vi "Controller VI.vi"(6 "Current Time In":u32, 7 "Read String":string, 8 "Down Detect Time In":u32, 9 "Up Detect Time In":u32, 10 "Left Detect Time In":u32, 11 "Right Detect Time In":u32) -> (0 "Down Detect Time Out":u32, 1 "Up Detect Time Out":u32, 2 "Left Detect Time Out":u32, 3 "Right detect Time Out":u32, 4 "Control Cluster":T1 {"Yaw Speed" scale=-1.0..1.0; "Vertical Speed" scale=-1.0..1.0; "Pitch" scale=-1.0..1.0; "Roll" scale=-1.0..1.0}, 5 "Command string":string)   [LabVIEW 2014]
uses:
  Others/Control cluster.ctl
  Global.vi
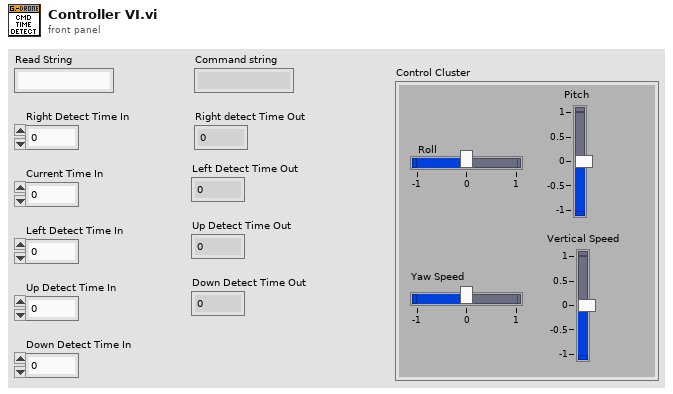
[diagram p1: front panel]
types:
  T1 = typedef "Control cluster.ctl" = cluster{"Roll":sgl, "Pitch":sgl, "Vertical Speed":sgl, "Yaw Speed":sgl}
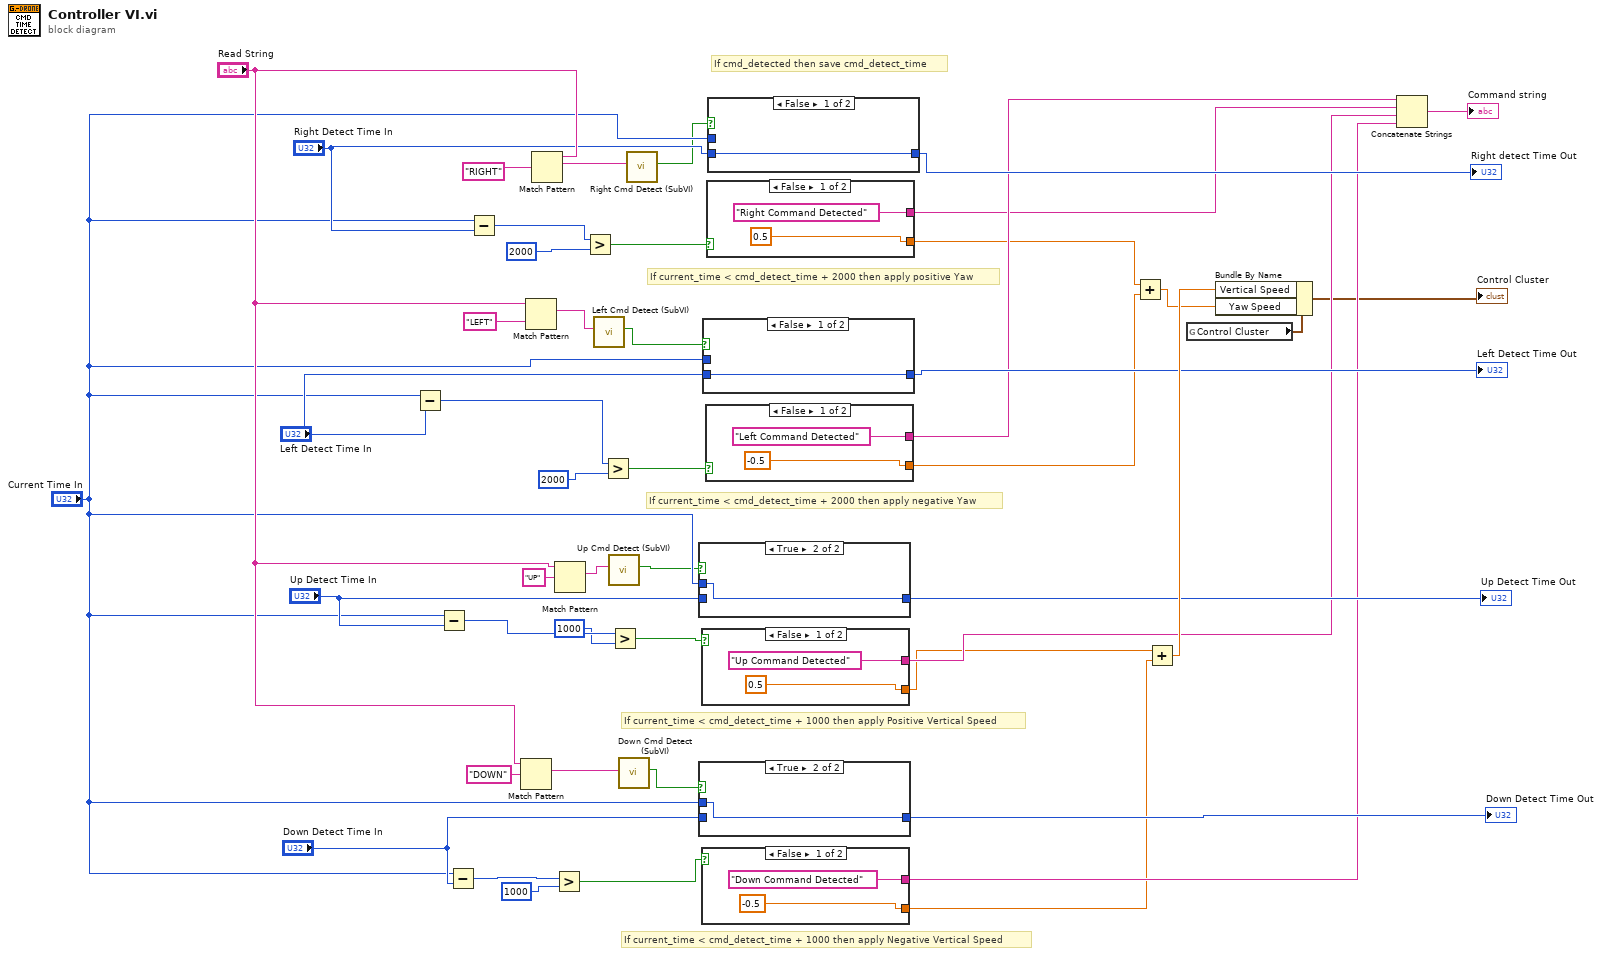
[diagram p0: block diagram]
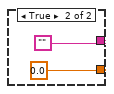
[diagram p2: hidden frame]
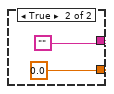
[diagram p4: hidden frame]
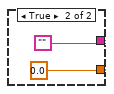
[diagram p6: hidden frame]
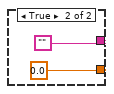
[diagram p8: hidden frame]
diagram:
  # "If current_time < cmd_detect_time + 1000 then apply Negative Vertical Speed"
  # "If current_time < cmd_detect_time + 1000 then apply Positive Vertical Speed"
  # "If current_time < cmd_detect_time + 2000 then apply negative Yaw"
  # "If cmd_detected then save cmd_detect_time"
  # "If current_time < cmd_detect_time + 2000 then apply positive Yaw"
  n1 = Subtract(x="Current Time In", y="Left Detect Time In") -> (x-y=w11:u32)
  n2 = Subtract(x="Current Time In", y="Up Detect Time In") -> (x-y=w19:u32)
  n3 = Subtract(x="Current Time In", y="Down Detect Time In") -> (x-y=w27:u32)
  n4 = Subtract(x="Current Time In", y="Right Detect Time In") -> (x-y=w3:u32)
  n5 = Match Pattern(string="Read String", regular expression="DOWN") -> (match substring=w31:string)  [unwired: 1 in, 3 out]
  n6 = Match Pattern(string="Read String", regular expression="LEFT") -> (match substring=w8:string)  [unwired: 1 in, 3 out]
  n7 = Match Pattern(string="Read String", regular expression="RIGHT") -> (match substring=w17:string)  [unwired: 1 in, 3 out]
  n8 = Greater?(x=w27, y=u32 1000) -> (0:w29:bool)
  n9 = Match Pattern(string="Read String", regular expression="UP") -> (match substring=w21:string)  [unwired: 1 in, 3 out]
  n10 = Greater?(x=w3, y=u32 2000) -> (0:w2:bool)
  n11 = call "Left Cmd Detect (SubVI).vi"("Read String"=w8) -> ("Left Command"=w9:bool)  [unwired: 10 in]
  n12 = Greater?(x=w11, y=u32 2000) -> (0:w12:bool)
  n13 = call "Up Cmd Detect (SubVI).vi"("Read String"=w21) -> ("Up Command"=w22:bool)  [unwired: 10 in]
  n14 = Greater?(x=w19, y=u32 1000) -> (0:w20:bool)
  n15 = call "Down Cmd Detect (SubVI).vi"("Read String"=w31) -> ("Down Command"=w30:bool)  [unwired: 10 in]
  n16 = call "Right Cmd Detect (SubVI).vi"("Read String"=w17) -> ("Right Command"=w16:bool)  [unwired: 10 in]
  n17 = case shown="True" w22 {
    tunnel: [w48 w49] -> w42
    tunnel: "Up Detect Time In" -> [w48 _]
    tunnel: "Current Time In" -> [_ w49]
    frame False {
    }
    frame True {
    }
  }
  "Up Detect Time Out" <- w42
  n18 = case shown="True" w30 {
    tunnel: [w50 w51] -> w37
    tunnel: "Down Detect Time In" -> [w50 _]
    tunnel: "Current Time In" -> [_ w51]
    frame False {
    }
    frame True {
    }
  }
  "Down Detect Time Out" <- w37
  n19 = case shown="False" w20 {
    tunnel: ["Up Command Detected" ""] -> w34
    tunnel: [0.5 0.0] -> w23
    frame False {
    }
    frame True {
    }
  }
  n20 = case shown="False" w29 {
    tunnel: ["Down Command Detected" ""] -> w33
    tunnel: [-0.5 0.0] -> w25
    frame False {
    }
    frame True {
    }
  }
  n21 = case shown="False" w9 {
    tunnel: [w60 w61] -> w41
    tunnel: "Left Detect Time In" -> [w60 _]
    tunnel: "Current Time In" -> [_ w61]
    frame False {
    }
    frame True {
    }
  }
  "Left Detect Time Out" <- w41
  n22 = case shown="False" w12 {
    tunnel: ["Left Command Detected" ""] -> w36
    tunnel: [-0.5 0.0] -> w14
    frame False {
    }
    frame True {
    }
  }
  n23 = case shown="False" w2 {
    tunnel: ["Right Command Detected" ""] -> w35
    tunnel: [0.5 0.0] -> w13
    frame False {
    }
    frame True {
    }
  }
  n24 = case shown="False" w16 {
    tunnel: [w70 w71] -> w43
    tunnel: "Right Detect Time In" -> [w70 _]
    tunnel: "Current Time In" -> [_ w71]
    frame False {
    }
    frame True {
    }
  }
  "Right detect Time Out" <- w43
  n25 = Add(x=w13, y=w14) -> (x+y=w15:dbl)
  n26 = Add(x=w23, y=w25) -> (x+y=w47:dbl)
  n27 = global read "Global.vi" "Control Cluster"() -> (w4:T1)
  n28 = Bundle By Name(cluster=w4, "Vertical Speed"=w47, "Yaw Speed"=w15) -> (→"Control Cluster":T1)
  n29 = Concatenate Strings(w36, w35, w34, w33) -> (→"Command string":string)
